vi "Write and Read Register.vi"() -> ()   [LabVIEW 2013]
panel:
  out "数字 2":u32
  out "子字符串 2":string
  out "数字":u32
  out "子字符串":string
  out "十六进制整型字符串":string
  out "x*y":u32 format="%x"
  out "ReadRegister":u32 format="%b"
  out "双精度浮点数":sgl
  in  "Write Reg Ref":u32 format="%x"
  in  "Write Value":u32
  in  "Write Reg!":bool
  in  "Read Reg!":bool
  in  "Read Register Ref":u32 format="%x"
  in  "Stop Grabbing":bool
  out "# of Iteration":i32
  in  "Live Image Display":refnum<k7>(container)
  # "This is an simlple ActiveX example using methods provided by ActiveFlyCapConctrol to grab images from an PGR camera,  \ndisplay it on the screen and retrieve the frame rate at the same time. Also, it can toggle between free running mode and software\ntrigger mode. It is meant to let new users become farmiliar with the ActiveX control provided by the Flycapture SDK, so more compilcated blocks can be build upon."
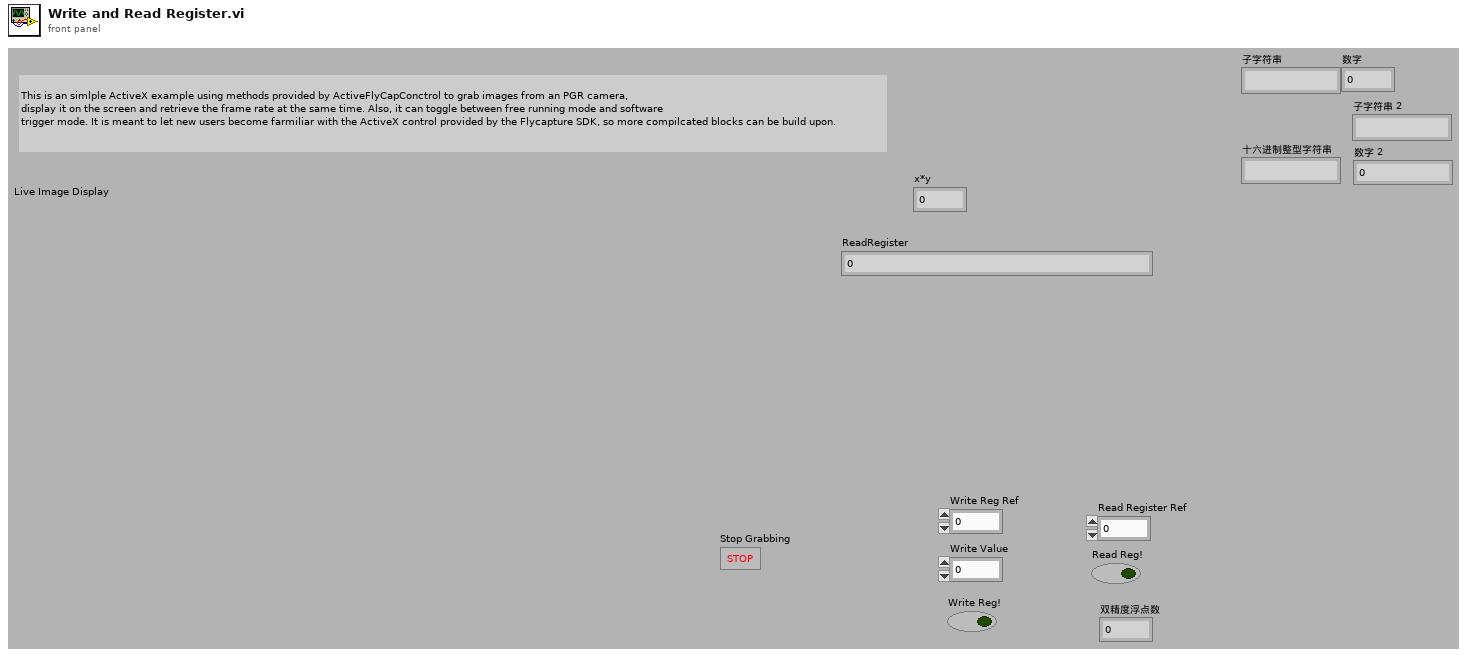
[diagram p1: front panel]
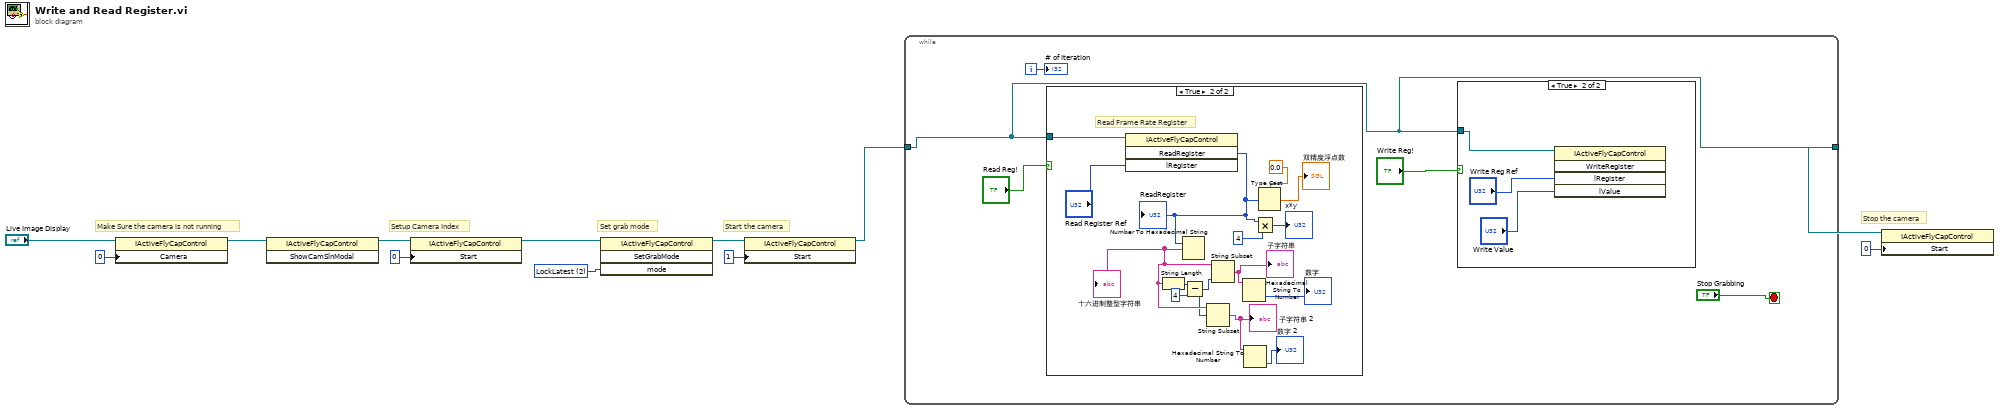
[diagram p0: block diagram]
diagram:
  w1 = 2 items=["FreeRunning", "LockNext", "LockLatest"] ("mode")
  # "Start the camera"
  # "Stop the camera"
  # "Setup Camera Index"
  # "Set grab mode"
  # "Make Sure the camera is not running"
  n1 = property class="IActiveFlyCapControl"(reference="Live Image Display", "Camera"=0 ("Start")) -> (reference out=w8:refnum<k7>)  [unwired: 1 in, 1 out]
  n2 = invoke class="IActiveFlyCapControl" method="ShowCamSlnModal"(reference=w8) -> (reference out=w7:refnum<k7>)  [unwired: 2 in, 2 out]
  n3 = property class="IActiveFlyCapControl"(reference=w7, "Start"=0 ("Camera")) -> (reference out=w9:refnum<k7>)  [unwired: 1 in, 1 out]
  n4 = invoke class="IActiveFlyCapControl" method="SetGrabMode"(reference=w9, "mode"=w1) -> (reference out=w2:refnum<k7>)  [unwired: 2 in, 3 out]
  n5 = property class="IActiveFlyCapControl"(reference=w2, "Start"=1) -> (reference out=w3:refnum<k7>)  [unwired: 1 in, 1 out]
  n6 = while {
    tunnel: w3 -> [w13]
    tunnel: [w13] -> w4
    i -> [w16]
    stop <- "Stop Grabbing" stop-if-true
    n7 = case shown="True" "Read Reg!" {
      tunnel: w13 -> [_ w35]
      frame False {
      }
      frame True {
        # "Read Frame Rate Register"
        n8 = invoke class="IActiveFlyCapControl" method="ReadRegister"(reference=w35, "lRegister"="Read Register Ref") -> ("ReadRegister"=w29:u32)  [unwired: 2 in, 3 out]
        "ReadRegister" <- w29
        n9 = Number To Hexadecimal String(2:w29) -> (0:w25:string)  [unwired: 1 in]
        "十六进制整型字符串" <- w25
        n10 = String Length(string=w25) -> (length=w28:i32)
        n11 = Subtract(x=w28, y=4) -> (x-y=w21:i32)
        n12 = String Subset(string=w25, offset (0)=w21) -> (substring=w23:string)  [unwired: 1 in]
        "子字符串 2" <- w23
        n13 = String Subset(string=w25, length (rest)=w21) -> (substring=w27:string)  [unwired: 1 in]
        "子字符串" <- w27
        n14 = Hexadecimal String To Number(string=w27) -> (number=→"数字":u32)  [unwired: 2 in, 1 out]
        n15 = Hexadecimal String To Number(string=w23) -> (number=→"数字 2":u32)  [unwired: 2 in, 1 out]
        n16 = Multiply(x=w29, y=u32 4) -> (x*y=→"x*y":u32)
        n17 = Type Cast(type=sgl 0.0 ("双精度浮点数"), x=w29) -> (*(type *) &x=→"双精度浮点数":sgl)
      }
    }
    n18 = case shown="True" "Write Reg!" {
      tunnel: w13 -> [_ w18]
      frame False {
      }
      frame True {
        n19 = invoke class="IActiveFlyCapControl" method="WriteRegister"(reference=w18, "lRegister"="Write Reg Ref", "lValue"="Write Value") -> ()  [unwired: 2 in, 5 out]
      }
    }
    "# of Iteration" <- w16
  }
  n20 = property class="IActiveFlyCapControl"(reference=w4, "Start"=0) -> ()  [unwired: 1 in, 2 out]
